vi "路径[2]-8.6.vi"(1 "输入路径":path) -> (0 "输出路径":path)   [LabVIEW 2013]
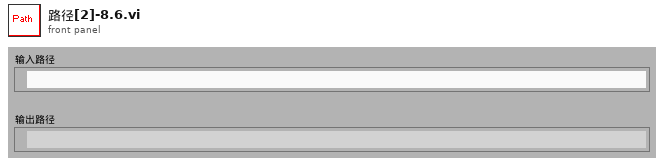
[diagram p1: front panel]
types:
  T1 = enum32{"invalid app kind", "Development System", "Run Time System", "Student Edition", "Embedded LabVIEW", "Evaluation", "Custom"}
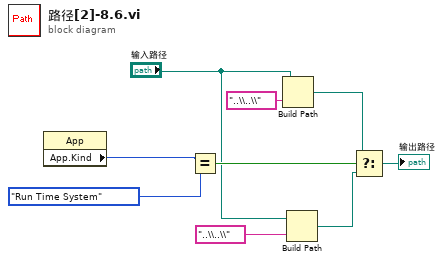
[diagram p0: block diagram]
diagram:
  n1 = property class="App"() -> ("App.Kind"=w9:T1)  [unwired: 2 in, 2 out]
  n2 = Equal?(x=w9, y=T1."Run Time System") -> (x = y?=w7:bool)
  n3 = Build Path(base path="输入路径", name or relative path="..\\..\\" ("名称或相对路径")) -> (appended path=w5:path)
  n4 = Build Path(base path="输入路径", name or relative path="..\\..\\" ("名称或相对路径")) -> (appended path=w6:path)
  n5 = Select(t=w5, s=w7, f=w6) -> (s? t:f=→"输出路径":path)
